vi "BRPOP.vi"(0 "refnum in":refnum<vi>, 1 "Keys":string[](array[string]), 5 "Timeout":string, 11 "error in":errorcluster) -> (4 "refnum out":refnum<vi>, 6 "Data":T1, 15 "error out":errorcluster)   [LabVIEW 2020]
uses:
  SubVIs/Controls/redis-data.ctl
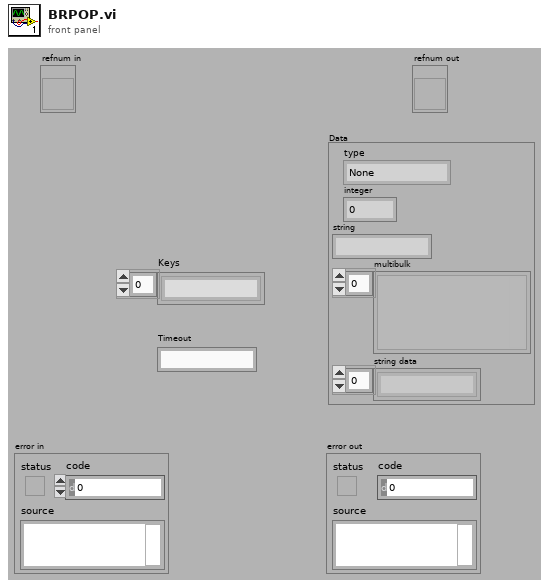
[diagram p1: front panel]
types:
  T1 = typedef "redis-data.ctl" = cluster{"type":enum16{"None", "Error", "Status", "Nil", "Integer", "String", "Multibulk"}, "integer":i64, "string":string, "multibulk":variant[], "string data":string[]}
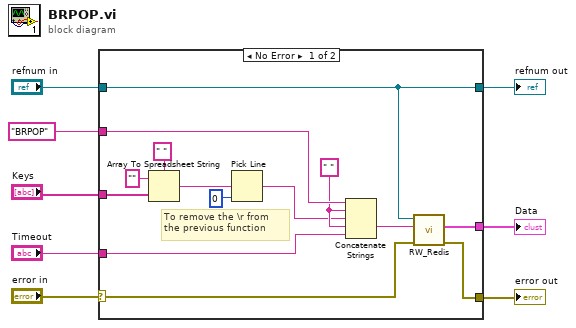
[diagram p0: block diagram]
diagram:
  n1 = case shown="No Error" "error in" {
    selector: "error in" -> [w16 w24]
    tunnel: "Keys" -> [w22 _]
    tunnel: "BRPOP" -> [w13 _]
    tunnel: "refnum in" -> [w11 w23]
    tunnel: [w15 w24] -> w5
    tunnel: [w14 _] -> w2
    tunnel: [w11 w23] -> w3
    tunnel: "Timeout" -> [w9 _]
    frame No Error {
      w12 = " "
      # "To remove the \\r from\nthe previous function"
      n2 = Array To Spreadsheet String(delimiter (Tab)=" ", array=w22, 3:"" ("format string")) -> (spreadsheet string=w19:string)
      n3 = Pick Line(multi-line string=w19, line index=0) -> (output string=w10:string)  [unwired: 1 in]
      n4 = Concatenate Strings(w13, w12, w10, w12, w9) -> (w17:string)
      n5 = call "RW_Redis.vi"("error in"=w16, "command"=w17, "refnum"=w11) -> ("error out"=w15:errorcluster, "Data"=w14:T1)  [unwired: 7 in]
    }
    frame Error {
    }
  }
  "error out" <- w5
  "refnum out" <- w3
  "Data" <- w2
